vi "List Contents of bucket.vi"() -> ()   [LabVIEW 2011]
doc: "This example shows you how to list the contents of your Amazon S3 bucket.\n\nThe list will contain information about all the objects you have in the bucket."
uses:
  Typedefs/Access_Key_Type.ctl
  Typedefs/Secret_Key_Type.ctl
  vi.lib/National Instruments/LabVIEW Interface for Amazon S3/Typedefs/AMZ_S3_AWS Credentials.ctl
  vi.lib/National Instruments/LabVIEW Interface for Amazon S3/LV Interface for Amazon S3.lvlib
panel:
  in  "Secret Key":T1
  in  "Access Key":T2
  in  "Bucket Contents":i32(listbox)
  # "To use this VI, you have to register first with Amazon to have an Amazon AWS account.\nIf you don't have an account yet, go to http://aws.amazon.com and Create an AWS account!"
  # "Note: You have to have some buckets created\nto see any effect after running this VI!\n1. Fill in your AWS Credentials\n2. Run this VI\n3. In the pop-up dialog select the bucket you\nwant to list"
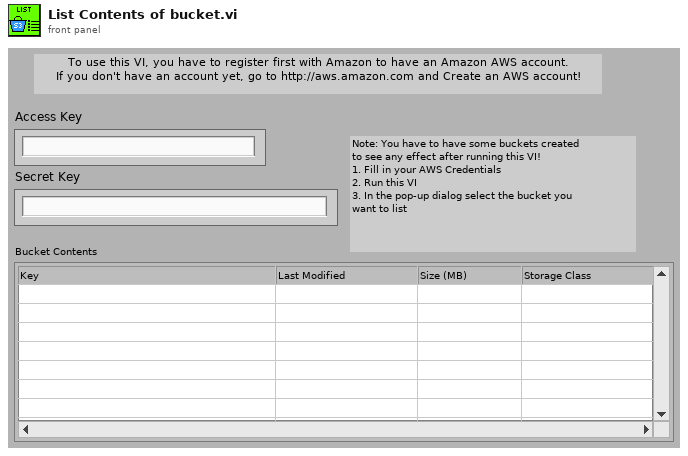
[diagram p1: front panel]
types:
  T1 = typedef "Secret_Key_Type.ctl" = string
  T2 = typedef "Access_Key_Type.ctl" = string
  T3 = typedef "LV Interface for Amazon S3.lvlib/AMZ_S3_AWS Credentials.ctl" = cluster{"Access Key":string, "Secret Key":string}
  T4 = typedef "LV Interface for Amazon S3.lvlib/AMZ_S3_API_Bucket.ctl" = cluster{"Name":string, "CreationDate":timestamp}
  T5 = typedef "LV Interface for Amazon S3.lvlib/AMZ_S3_API_ListBucketResult Content.ctl" = cluster{"Key":string, "LastModified":timestamp, "ETag":string, "Size":u64, "Storage Class":T6, "Owner":T7}
  T6 = typedef "LV Interface for Amazon S3.lvlib/AMZ_S3_Storage Class.ctl" = enum16{"STANDARD", "REDUCED_REDUNDANCY"}
  T7 = typedef "LV Interface for Amazon S3.lvlib/AMZ_S3_API_Owner.ctl" = cluster{"ID":string, "DisplayName":string}
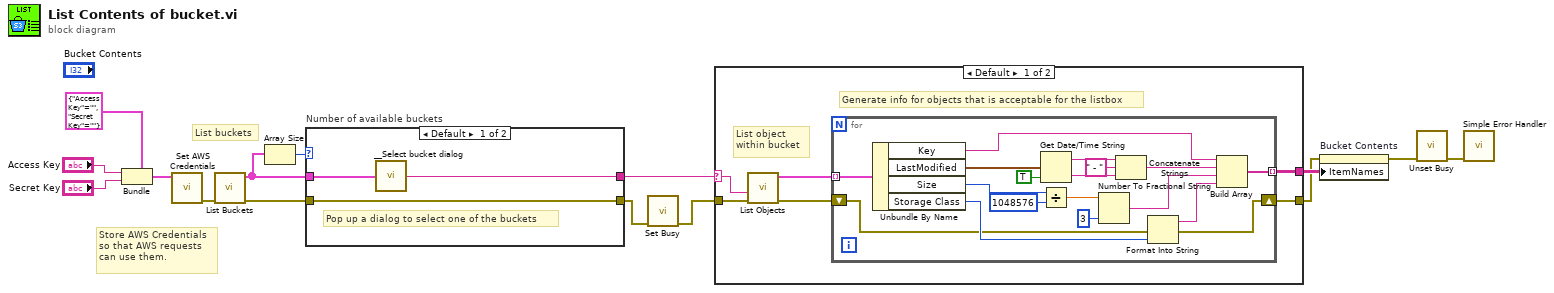
[diagram p0: block diagram]
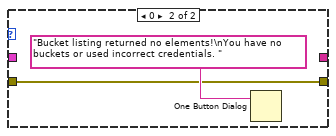
[diagram p3: hidden frame]
diagram:
  # "List buckets"
  # "Store AWS Credentials\nso that AWS requests\ncan use them."
  n1 = Bundle(cluster=T3 {"Access Key"="", "Secret Key"=""} ("AWS Credentials in"), "Access Key"="Access Key", "Secret Key"="Secret Key") -> (w1:T3)
  n2 = call "Set AWS Credentials.vi"("AWS Credentials in"=w1) -> ("error out"=w15:errorcluster)  [unwired: 10 in]
  n3 = call "List Buckets.vi"("error in (no error)"=w15) -> ("error out"=w9:errorcluster, "Buckets"=w13:T4[])  [unwired: 9 in]
  n4 = Array Size(array=w13) -> (size(s)=w14:i32)
  n5 = case "Number of available buckets" shown="Default" w14 {
    tunnel: w13 -> [w18 _]
    tunnel: [w17 _] -> w12
    tunnel: w9 -> [w16 w19]
    tunnel: [w16 w19] -> w8
    frame Default {
      # "Pop up a dialog to select one of the buckets"
      n6 = call "__Select bucket dialog.vi"("Buckets"=w18) -> ("Selected bucket"=w17:string)
    }
    frame 0 {
      n7 = One Button Dialog(message="Bucket listing returned no elements!\nYou have no buckets or used incorrect credentials. ") -> ()  [unwired: 1 in, 1 out]
    }
  }
  n8 = call <vilib>:"Set Busy.vi"("error in (no error)"=w8) -> ("error out"=w7:errorcluster)  [unwired: 9 in, 1 out]
  n9 = case shown="Default" w12 {
    selector: w12 -> [w26 _]
    tunnel: w7 -> [w25 w45]
    tunnel: [w22 _] -> w11
    tunnel: [w21 w45] -> w10
    frame Default {
      # "Generate info for objects that is acceptable for the listbox"
      # "List object\nwithin bucket"
      n10 = call "List Objects.vi"("error in (no error)"=w25, "Bucket"=w26) -> ("error out"=w23:errorcluster, "Contents"=w24:T5[])  [unwired: 8 in]
      n11 = for {
        tunnel: w24 -> [w44] mode=indexing
        shift-right: [w28] -> w21
        shift-left: w23 -> [w29]
        tunnel: [w27] -> w22 mode=indexing
        n12 = Unbundle By Name(w44) -> ("Key"=w33:string, "LastModified"=w35:timestamp, "Size"=w43:u64, "Storage Class"=w34:T6)
        n13 = Get Date/Time String(seconds (now)=w35, want seconds? (F)=TRUE) -> (date string=w38:string, time string=w37:string)  [unwired: 1 in]
        n14 = Divide(x=w43, y=u64 1048576) -> (x/y=w41:dbl)
        n15 = Number To Fractional String(number=w41, precision (6)=i16 3) -> (F-format string=w31:string)  [unwired: 2 in]
        n16 = Concatenate Strings(w38, " - " ("string"), w37) -> (w32:string)
        n17 = Format Into String(error in=w29, w34) -> (resulting string=w30:string, error out=w28:errorcluster)  [unwired: 2 in]
        n18 = Build Array(w33, w32, w31, w30) -> (w27:string[])
      }
    }
    frame "" {
      # "No bucket selected, do nothing"
    }
  }
  n19 = property on="Bucket Contents" class="MCListbox (strict)"(error in=w10, "ItemNames"=w11) -> (error out=w6:errorcluster)  [unwired: 1 in, 1 out]
  n20 = call <vilib>:"Unset Busy.vi"("error in (no error)"=w6) -> ("error out"=w5:errorcluster)  [unwired: 10 in]
  n21 = call <vilib>:"Simple Error Handler.vi"("error in (no error)"=w5) -> ()  [unwired: 4 in, 5 out]
